vi "Vision Calculations.vi"(0 "Image In":T2, 3 "error in":errorcluster) -> (5 "Vision Data":T1)   [LabVIEW 2014]
uses:
  <vilib>/vision/Image Controls.llb/IMAQ Image.ctl
  typedefs/vision/vision data.ctl
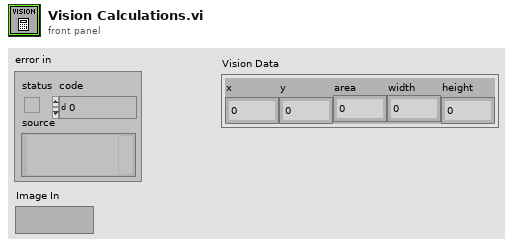
[diagram p1: front panel]
types:
  T1 = typedef "vision data.ctl" = cluster{"x":dbl, "y":dbl, "area":dbl, "width":dbl, "height":dbl}
  T2 = typedef "IMAQ Image.ctl" = refnum<image>
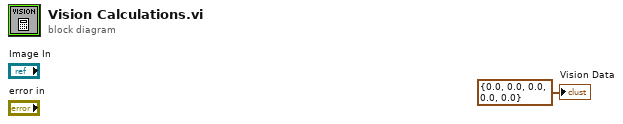
[diagram p0: block diagram]
diagram:
  "Vision Data" <- T1 {"x"=0.0, "y"=0.0, "area"=0.0, "width"=0.0, "height"=0.0} ("Vision Data")
